vi "Werte ueber Sekunden mitteln.vi"(0 "Neuer Wert":sgl, 7 "Sek":u32, 11 "error in (no error)":errorcluster caption="Fehler (Eingang, kein Fehler)") -> (4 "gemittelter Wert":sgl, 15 "error out":errorcluster caption="Fehler (Ausgang)")   [LabVIEW 2020, in "allgemeine Sub-VIs.lvlib"]
uses:
  allgemeine Sub-VIs.lvlib
  Seiten/FT-IR/Aktionen EVID-Codes.ctl
  Seiten/FT-IR/FGV FT-IR Aktionen.ctl
  Seiten/FT-IR/FT-IR.lvlib
panel:
  # "Ablaufinvariante Ausführung"
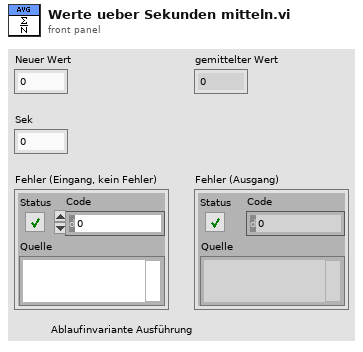
[diagram p1: front panel]
types:
  T1 = typedef "FT-IR.lvlib/FGV FT-IR Aktionen.ctl" = enum16{"lesen", "NOG setzen", "NOS setzen", "Initialisieren", "speichern", "ALLES setzen", "FT-IR Spektrum loggen", "Komm Stoppen", "Spektrum LogKonfig"}
  T2 = typedef "FT-IR.lvlib/Aktionen EVID-Codes.ctl" = enum16{"lesen", "setzen", "laden", "speichern", "1Hz/5Hz", "Smoothing", "Rolling Average"}
  T3 = typedef "FT-IR.lvlib/1Hz-5Hz Geraet.ctl" = u16
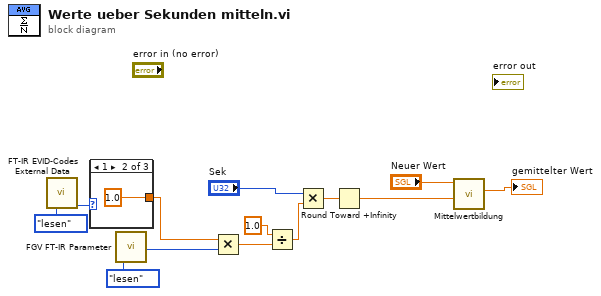
[diagram p0: block diagram]
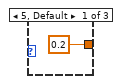
[diagram p2: hidden frame]
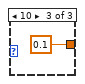
[diagram p3: hidden frame]
diagram:
  n1 = call "FT-IR EVID-Codes External Data.vi"("Aktionen"=Aktionen_EVID-Codes."lesen") -> ("1Hz/5Hz Gerät"=w7:T3)  [unwired: 9 in, 5 out]
  n2 = case shown="1" w7 {
    tunnel: [0.2 1.0 0.1] -> w4
    frame 5, Default {
    }
    frame 1 {
    }
    frame 10 {
    }
  }
  n3 = call "FGV FT-IR Parameter.vi"("Aktion"=FGV_FT-IR_Aktionen."lesen") -> ("NoOfScan"=w5:u32)  [unwired: 11 in, 7 out]
  n4 = Multiply(x=w4, y=w5) -> (x*y=w12:dbl)
  n5 = Divide(x=1.0, y=w12) -> (x/y=w9:dbl)
  n6 = Multiply(x="Sek", y=w9) -> (x*y=w11:dbl)
  n7 = Round Toward +Infinity(x=w11) -> (ceil(x): smallest int >= x=w3:dbl)
  n8 = call "Mittelwertbildung.vi"("Anzahl Werte"=w3, "Neuer Wert"="Neuer Wert") -> ("gemittelter Wert"=→"gemittelter Wert":sgl)  [unwired: 7 in, 2 out]
